vi "writeDelay.vi"(8 "error in (no error)":errorcluster, 10 "Delay(us)":u32, 11 "ModbusBuffer in":refnum<class "ModbusBuffer.lvclass">) -> (0 "error out":errorcluster, 3 "ModbusBuffer out":refnum<class "ModbusBuffer.lvclass">)   [LabVIEW 2016, in "RTModbus.lvlib" / "ModbusBuffer.lvclass"]
uses:
  ModbusBuffer.lvclass
  ModbusBuffer.lvclass/ModbusBuffer.ctl
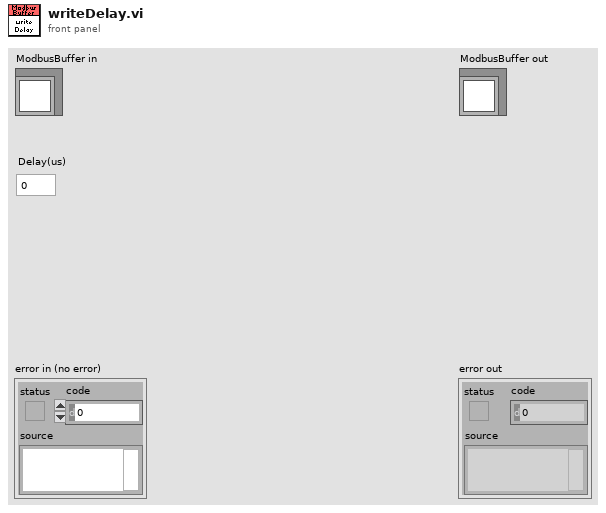
[diagram p1: front panel]
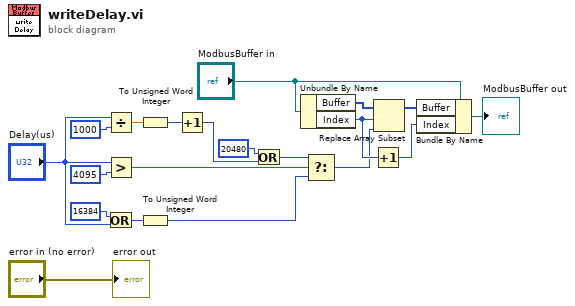
[diagram p0: block diagram]
diagram:
  n1 = Divide(x="Delay(us)", y=u32 1000) -> (x/y=w18:dbl)
  n2 = Greater?(x="Delay(us)", y=u32 4095) -> (0:w16:bool)
  n3 = Or(x=u16 16384, y="Delay(us)") -> (x .or. y?=w4:u32)
  n4 = To Unsigned Word Integer(number=w18) -> (unsigned 16bit integer=w15:u16)
  n5 = To Unsigned Word Integer(number=w4) -> (unsigned 16bit integer=w17:u16)
  n6 = Increment(x=w15) -> (x+1=w3:u16)
  n7 = Or(x=u16 20480, y=w3) -> (x .or. y?=w1:u16)
  n8 = Unbundle By Name("ModbusBuffer in") -> ("Buffer"=w14:u16[], "Index"=w10:i32)
  n9 = Select(t=w1, s=w16, f=w17) -> (s? t:f=w7:u16)
  n10 = Increment(x=w10) -> (x+1=w9:i32)
  n11 = Replace Array Subset(array=w14, new element=w7, index=w10) -> (w11:u16[])
  n12 = Bundle By Name(cluster="ModbusBuffer in", "Buffer"=w11, "Index"=w9) -> (→"ModbusBuffer out":refnum<class "ModbusBuffer.lvclass">)
  "error out" <- "error in (no error)"
